vi "VerifConfigState.vi"(8 "error in (no error)":errorcluster, 11 "Acquisition in":refnum<class "Acquisition.lvclass">) -> (0 "error out":errorcluster, 3 "Acquisition out":refnum<class "Acquisition.lvclass">)   [LabVIEW 2018, in "Acquisition.lvclass"]
uses:
  Acquisition.lvclass
  Acquisition.lvclass/Acquisition.ctl
  Channel/Channel.lvclass
  StateMachine/State Machine.lvclass
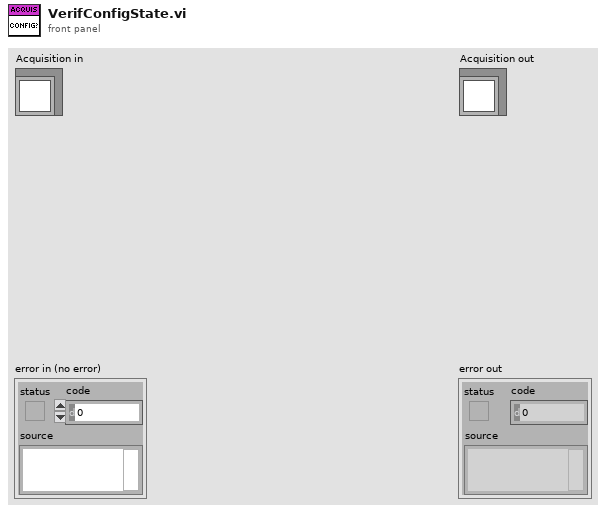
[diagram p1: front panel]
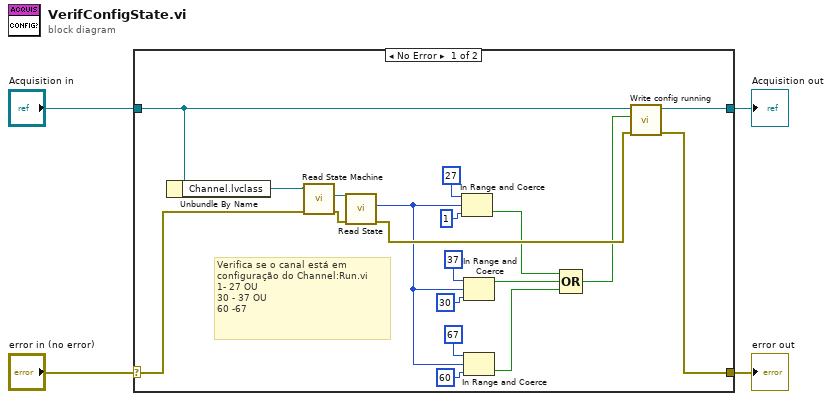
[diagram p0: block diagram]
diagram:
  n1 = case shown="No Error" "error in (no error)" {
    selector: "error in (no error)" -> [w19 w25]
    tunnel: [w14 w25] -> w3
    tunnel: [w16 w24] -> w1
    tunnel: "Acquisition in" -> [w17 w24]
    frame No Error {
      # "Verifica se o canal está em \nconfiguração do Channel:Run.vi\n1- 27 OU\n30 - 37 OU\n60 -67"
      n2 = Unbundle By Name(w17) -> ("Channel.lvclass"=w20:refnum<class "Channel.lvclass">)
      n3 = call-dynamic "Read State Machine.vi"("error in (no error)"=w19, "Device in"=w20) -> ("error out"=w18:errorcluster, "State Machine.lvclass"=w23:refnum<class "State Machine.lvclass">)  [unwired: 7 in, 1 out]
      n4 = call-dynamic "Read State.vi"("error in (no error)"=w18, "State Machine in"=w23) -> ("error out"=w15:errorcluster, "State"=w5:i32)  [unwired: 7 in, 1 out]
      n5 = In Range and Coerce(upper limit=27, x=w5, lower limit=1) -> (In Range?=w9:bool)  [unwired: 1 out]
      n6 = In Range and Coerce(upper limit=37, x=w5, lower limit=30) -> (In Range?=w8:bool)  [unwired: 1 out]
      n7 = In Range and Coerce(upper limit=67, x=w5, lower limit=60) -> (In Range?=w7:bool)  [unwired: 1 out]
      n8 = Compound Arithmetic op=OR(w9, w8, w7) -> (w6:bool)
      n9 = call-dynamic "Write config running.vi"("error in (no error)"=w15, "config running"=w6, "Server in"=w17) -> ("error out"=w14:errorcluster, "Server out"=w16:refnum<class "Acquisition.lvclass">)  [unwired: 7 in]
    }
    frame Error {
    }
  }
  "error out" <- w3
  "Acquisition out" <- w1
